vi "Analog_Begin.vi"   [LabVIEW 2014]
uses:
  <vilib>/Rock Robotics/SystemInterfaces/AI/FPGA_AIChannel.ctl
panel:
  # "e"
types:
  T1 = typedef "FPGA_AIChannel.ctl" = enum8{"AI 0", "AI 1", "AI 2", "AI 3", "AI MXP 0", "AI MXP 1", "AI MXP 2", "AI MXP 3", "Invalid"}
  T2 = typedef "WPI_AnalogChannelDevRef.ctl" = cluster{"DevStatus":errorcluster, "Controller":T3, "Analog Channel":T1}
  T3 = typedef "FPGA_TypedefAnalogModule.ctl" = enum16{"Controller 1"}
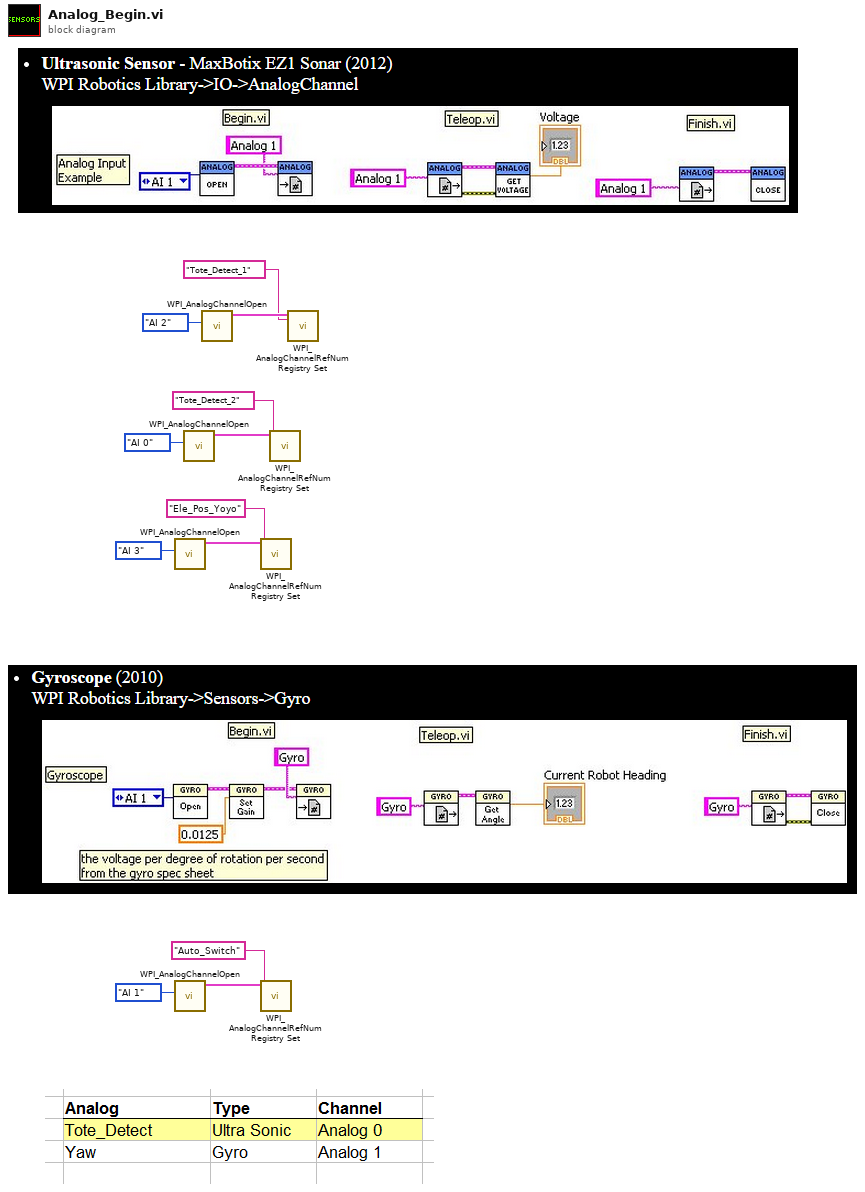
[diagram p0: block diagram]
diagram:
  n1 = call <vilib>:"WPI_AnalogChannelOpen.vi"("Analog Channel"=FPGA_AIChannel."AI 3") -> ("AIDeviceRef"=w8:T2)  [unwired: 9 in, 1 out]
  n2 = call <vilib>:"WPI_AnalogChannelOpen.vi"("Analog Channel"=FPGA_AIChannel."AI 1") -> ("AIDeviceRef"=w2:T2)  [unwired: 9 in, 1 out]
  n3 = call <vilib>:"WPI_AnalogChannelOpen.vi"("Analog Channel"=FPGA_AIChannel."AI 0") -> ("AIDeviceRef"=w11:T2)  [unwired: 9 in, 1 out]
  n4 = call <vilib>:"WPI_AnalogChannelOpen.vi"("Analog Channel"=FPGA_AIChannel."AI 2") -> ("AIDeviceRef"=w6:T2)  [unwired: 9 in, 1 out]
  n5 = call <vilib>:"WPI_AnalogChannelRefNum Registry Set.vi"("refnum name"="Ele_Pos_Yoyo", "AIDeviceRef"=w8) -> ()  [unwired: 8 in, 2 out]
  n6 = call <vilib>:"WPI_AnalogChannelRefNum Registry Set.vi"("refnum name"="Auto_Switch", "AIDeviceRef"=w2) -> ()  [unwired: 8 in, 2 out]
  n7 = call <vilib>:"WPI_AnalogChannelRefNum Registry Set.vi"("refnum name"="Tote_Detect_2", "AIDeviceRef"=w11) -> ()  [unwired: 8 in, 2 out]
  n8 = call <vilib>:"WPI_AnalogChannelRefNum Registry Set.vi"("refnum name"="Tote_Detect_1", "AIDeviceRef"=w6) -> ()  [unwired: 8 in, 2 out]
